vi "Set Average Time.vi"(7 "error in":errorcluster {"code" format="%.0x"}, 9 "Assign  averexp according to the chart on the right":dbl=4.0, 10 "VISA resource name":refnum<visa-resource-name>="GPIB12::28::INSTR") -> (0 "error out":errorcluster {"code" format="%.0x"}, 1 "Read out result":string, 2 "Send string":string, 3 "VISA resource name out":refnum<visa-resource-name>)   [LabVIEW 2019, in "AH2500A.lvclass"]
uses:
  AH2500A.lvclass
panel:
  in  "byte count":u32=128
  # "Average over time: setting the measurement time"
  # "Default setting is 4"
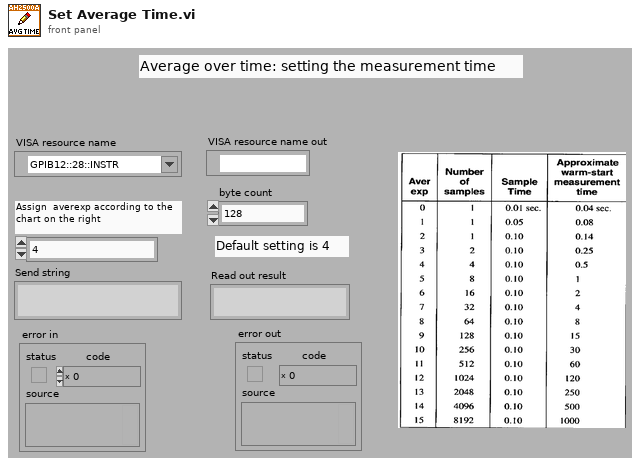
[diagram p1: front panel]
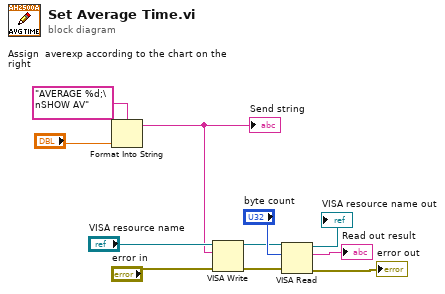
[diagram p0: block diagram]
diagram:
  n1 = Format Into String(format string="AVERAGE %d;\nSHOW AV", "Assign  averexp according to the chart on the right") -> (resulting string=w1:string)  [unwired: 2 in, 1 out]
  "Send string" <- w1
  n2 = VISA Write(VISA resource name="VISA resource name", write buffer=w1, error in (no error)="error in") -> (VISA resource name out=w5:refnum<visa-resource-name>, error out=w4:errorcluster)  [unwired: 1 out]
  n3 = VISA Read(VISA resource name=w5, byte count="byte count", error in (no error)=w4) -> (VISA resource name out=→"VISA resource name out":refnum<visa-resource-name>, read buffer=→"Read out result":string, error out=→"error out":errorcluster)  [unwired: 1 out]
